vi "动力环境监测系统.vi"() -> ()   [LabVIEW 2016]
uses:
  DAM0404D/DAM0404D/DAM0404D.lvclass
  C:/Program Files (x86)/National Instruments/LabVIEW 2016/vi.lib/ActorFramework/Actor/Actor.lvclass
  DAM0404D/DAM0404D/DAM0404D.lvclass/DAM0404D.ctl
  <vilib>/ActorFramework/Message Enqueuer/Message Enqueuer.lvclass/Message Enqueuer.ctl
  DAM0404D/DAM0404D Messages/Write Coil Msg/Write Coil Msg.lvclass/Write Coil Msg.ctl
  <vilib>/ActorFramework/Message Enqueuer/Enqueue.vi
  <vilib>/ActorFramework/Stop Msg/Stop Msg.lvclass
  C:/Program Files (x86)/National Instruments/LabVIEW 2016/vi.lib/ActorFramework/Message/Message.lvclass
  DAM0404D/DAM0404D Messages/Close MB Msg/Close MB Msg.lvclass
  DAM0404D/DAM0404D Messages/Open MB Msg/Open MB Msg.lvclass
  DAM0404D/DAM0404D Messages/Write Coil Msg/Write Coil Msg.lvclass
  DAM0404D/DAM0404D Messages/Read sTA Msg/Read sTA Msg.lvclass
  <vilib>/ActorFramework/Message Priority Queue/Priority Enqueue.vi
  <vilib>/ActorFramework/Actor/Actor.lvclass
  <vilib>/Utility/config.llb/NI_LVConfig.lvlib
panel:
  in  "Log":string
  out "Busy":bool
  in  "Boolean":bool
  in  "断电":bool
  in  "通电":bool
  out "Array":bool[](array[boolean])
  in  "串口打开":bool
  in  "VISA resource name":refnum<visa-resource-name>
  # "254：9600"
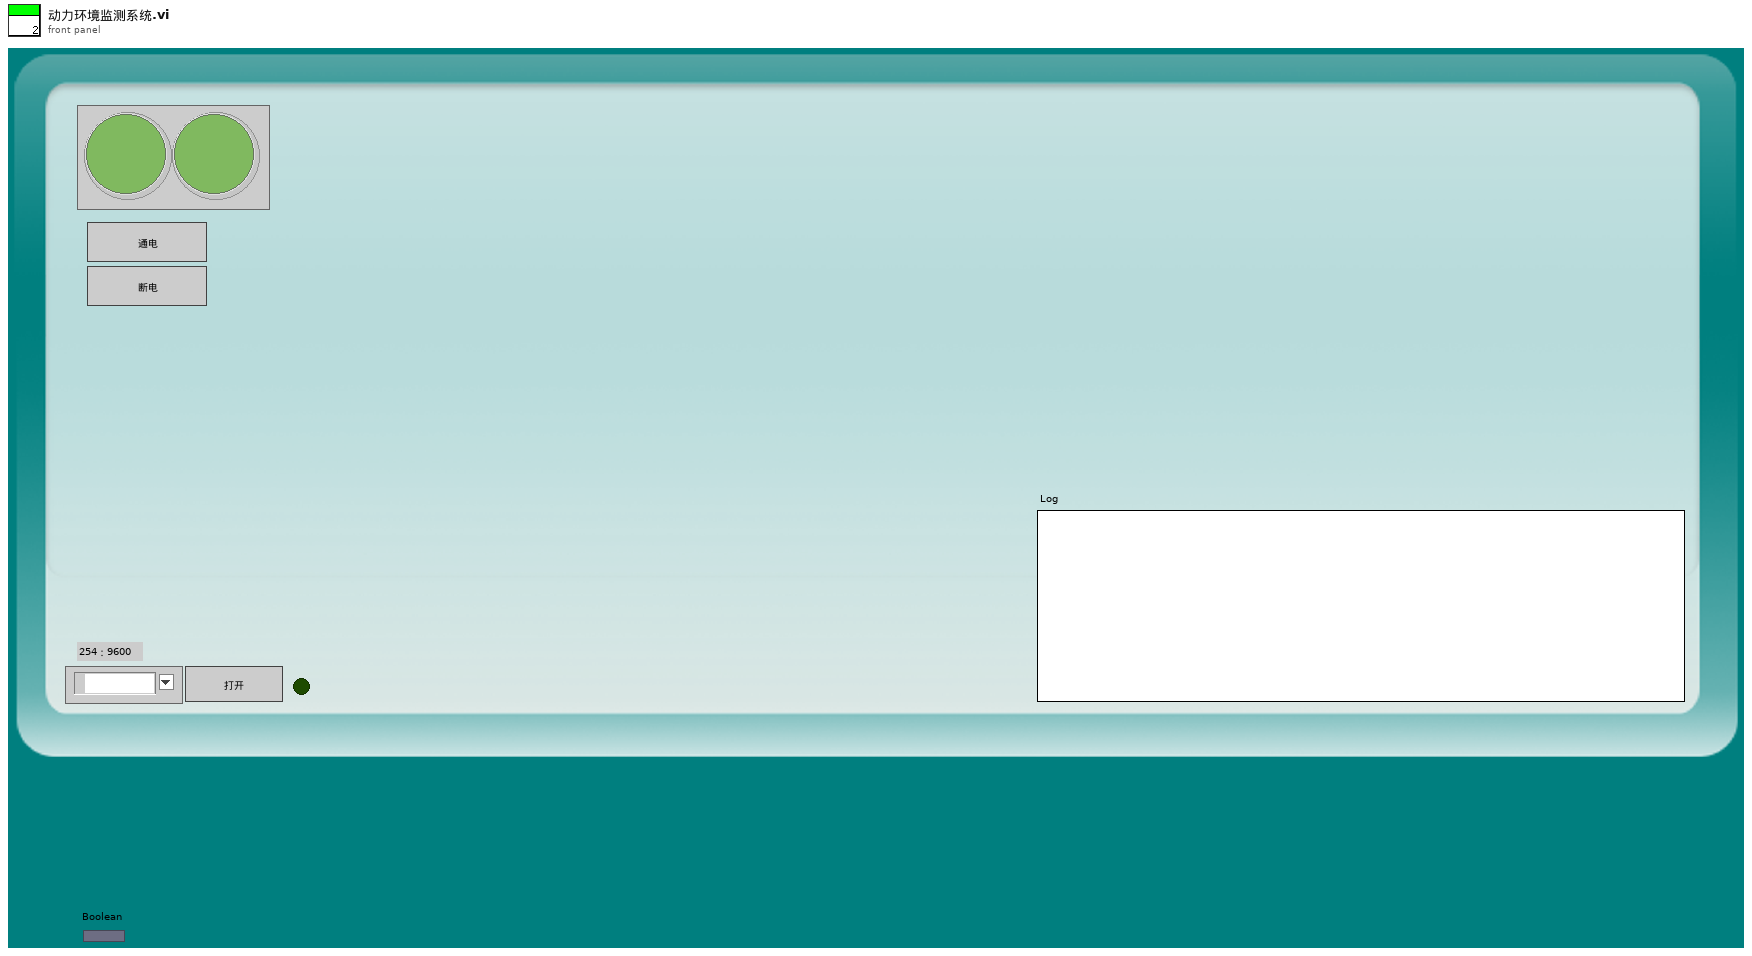
[diagram p1: front panel]
types:
  T1 = enum8{"Enabled", "Disabled", "Disabled and Grayed Out"}
  T2 = typedef "NI_LVConfig.lvlib/Config Data RefNum.ctl" = refnum<k1>
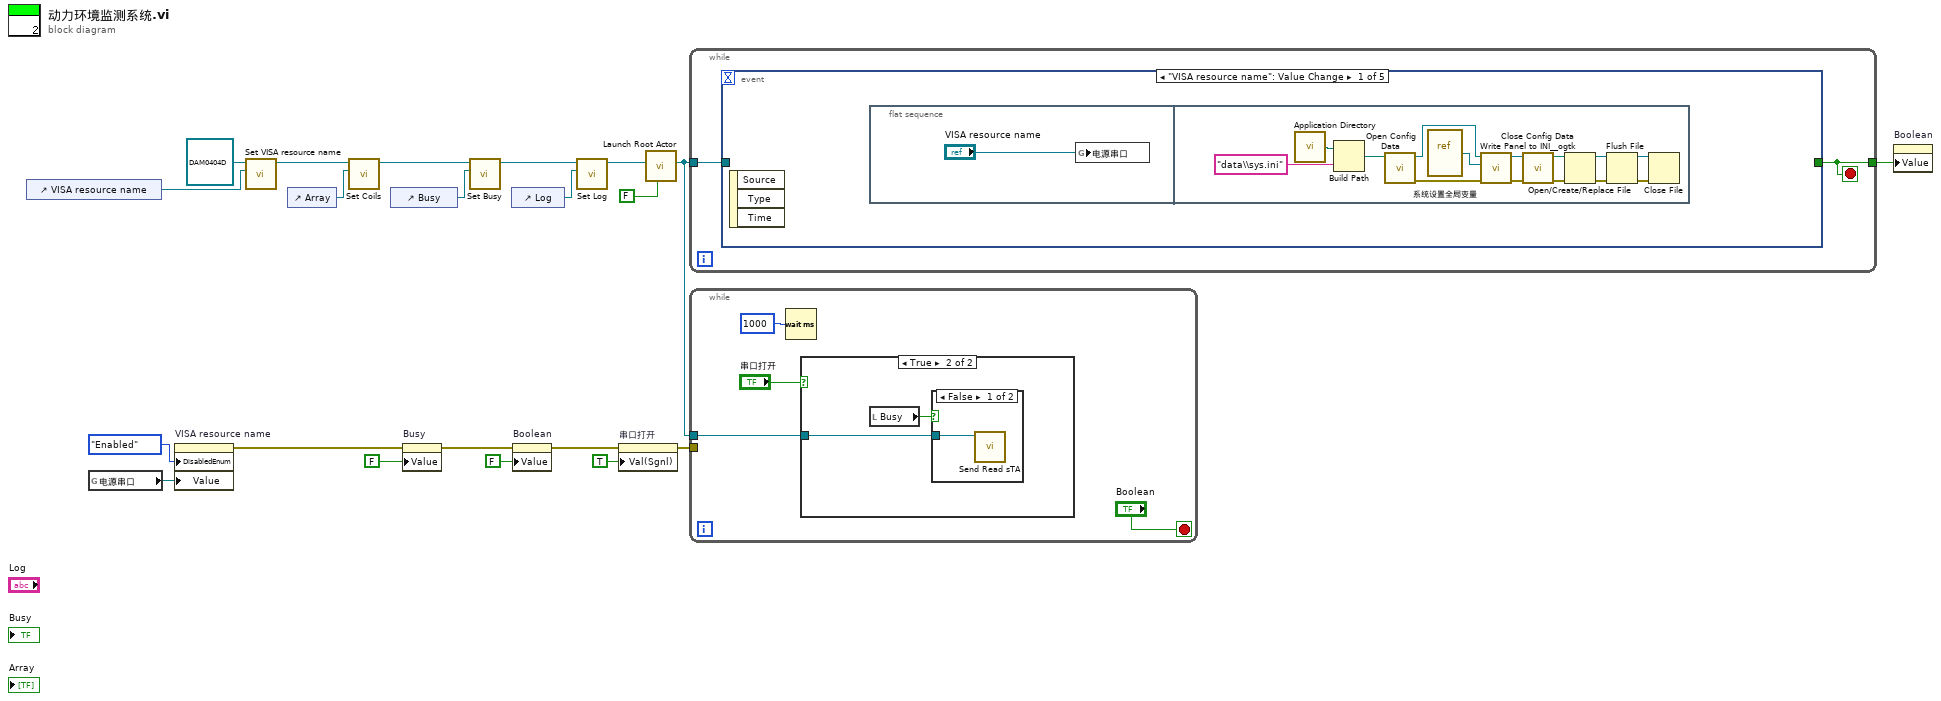
[diagram p0: block diagram]
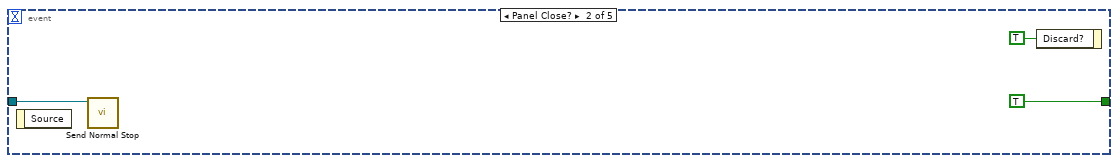
[diagram p4: hidden frame]
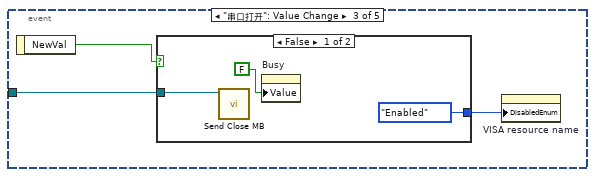
[diagram p5: hidden frame]
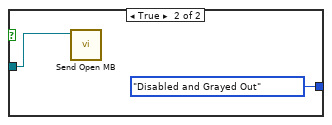
[diagram p6: hidden frame]
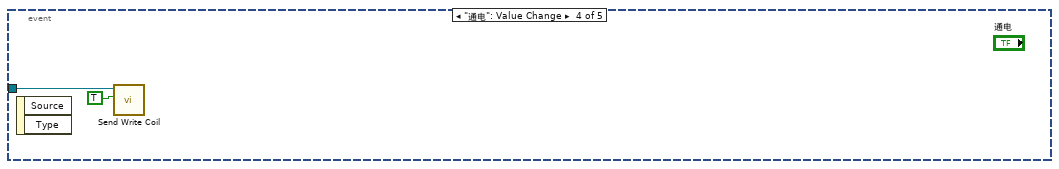
[diagram p7: hidden frame]
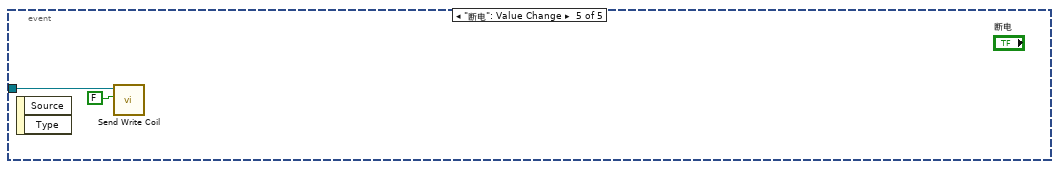
[diagram p8: hidden frame]
diagram:
  n1 = control-ref of="VISA resource name"() -> (w5:refnum<vi>)
  n2 = global read "系统设置全局变量.vi" "电源串口"() -> (w4:refnum<visa-resource-name>)
  n3 = property on="VISA resource name" class="VISAName"("DisabledEnum"=T1."Enabled" ("Disabled"), "Value"=w4) -> (error out=w10:errorcluster)  [unwired: 2 in, 1 out]
  n4 = call "Set VISA resource name.vi"("VISA resource name"=w5, "DAM0404D in"=refnum<class "DAM0404D.lvclass"> refnum ("DAM0404D.lvlib:DAM0404D.lvclass")) -> ("DAM0404D out"=w20:refnum<class "DAM0404D.lvclass">)  [unwired: 9 in]
  n5 = control-ref of="Array"() -> (w19:refnum<vi>)
  n6 = call "Set Coils.vi"("Coils"=w19, "DAM0404D in"=w20) -> ("DAM0404D out"=w14:refnum<class "DAM0404D.lvclass">)  [unwired: 9 in]
  n7 = control-ref of="Busy"() -> (w13:refnum<vi>)
  n8 = property on="Busy" class="Bool (strict)"(error in=w10, "Value"=FALSE ("Busy")) -> (error out=w12:errorcluster)  [unwired: 1 in, 1 out]
  n9 = call "Set Busy.vi"("Busy"=w13, "DAM0404D in"=w14) -> ("DAM0404D out"=w8:refnum<class "DAM0404D.lvclass">)  [unwired: 9 in]
  n10 = control-ref of="Log"() -> (w6:refnum<vi>)
  n11 = property on="Boolean" class="Bool (strict)"(error in=w12, "Value"=FALSE ("Boolean")) -> (error out=w3:errorcluster)  [unwired: 1 in, 1 out]
  n12 = call "Set Log.vi"("Log"=w6, "DAM0404D in"=w8) -> ("DAM0404D out"=w7:refnum<class "DAM0404D.lvclass">)  [unwired: 9 in]
  n13 = property on="串口打开" class="Bool (strict)"(error in=w3, "Val(Sgnl)"=TRUE ("Value (Signaling)")) -> (error out=w2:errorcluster)  [unwired: 1 in, 1 out]
  n14 = call <vilib>:"Launch Root Actor.vi"("Open Actor Core front panel? (F)"=FALSE, "Actor"=w7) -> ("Actor's Enqueuer"=w17:refnum<class "Message Enqueuer.lvclass">)  [unwired: 8 in, 1 out]
  n15 = while {
    tunnel: w17 -> [w23]
    tunnel: [w22] -> w18
    stop <- w22 stop-if-true
    n16 = event shown="[0] \"VISA resource name\": Value Change" {
      selector: _ -> [_ _ _ _ _]
      dyn-events: _ -> [_ _ _ _ _]
      timeout: _ -> [_ _ _ _ _]
      tunnel: [_ TRUE _ _ _] -> w22
      tunnel: w23 -> [_ w39 w44 w51 w53]
      event "VISA resource name": Value Change {
        n17 = event-data() -> ()  [unwired: 1 in, 3 out]
        n18 = flat-sequence {
          frame #0 {
            n19 = global write "系统设置全局变量.vi" "电源串口"("VISA resource name") -> ()
          }
          frame #1 {
            n20 = call <vilib>:"Application Directory.vi"() -> ("Application Directory"=w38:path)
            n21 = Build Path(base path=w38, name or relative path="data\\sys.ini" ("名称或相对路径")) -> (appended path=w36:path)
            n22 = call <vilib>:"Open Config Data.vi"("configuration file path"=w36) -> ("error out"=w32:errorcluster, "refnum"=w35:T2)  [unwired: 8 in, 1 out]
            n23 = vi-ref "系统设置全局变量.vi"() -> (w34:refnum<vi>)
            n24 = call <userlib>:"Write Panel to INI__ogtk.vi"("error in (no error)"=w32, "VI ref"=w34, "refnum"=w35) -> ("error out"=w31:errorcluster, "refnum out"=w33:T2)  [unwired: 7 in]
            n25 = call <vilib>:"Close Config Data.vi"("error in (no error)"=w31, "refnum"=w33) -> ("error out"=w26:errorcluster, "file path"=w25:path)  [unwired: 8 in]
            n26 = Open/Create/Replace File(file path (use dialog)=w25, error in=w26) -> (refnum out=w29:refnum<file>, error out=w30:errorcluster)  [unwired: 4 in, 1 out]
            n27 = Flush File(refnum=w29, error in=w30) -> (refnum out=w28:refnum<file>, error out=w27:errorcluster)
            n28 = Close File(refnum=w28, error in=w27) -> ()  [unwired: 2 out]
          }
        }
      }
      event Panel Close? {
        n29 = event-data() -> ()  [unwired: 1 in, 1 out]
        n30 = call <vilib>:"Send Normal Stop.vi"("Message Enqueuer"=w39) -> ()  [unwired: 10 in, 1 out]
        n31 = event-data("Discard?"=TRUE) -> ()  [unwired: 1 in, 1 out]
      }
      event "串口打开": Value Change {
        n32 = event-data() -> ("NewVal"=w43:bool)  [unwired: 1 in]
        n33 = case shown="False" w43 {
          tunnel: w44 -> [w46 w49]
          tunnel: [T1."Enabled" ("Disabled") T1."Disabled and Grayed Out" ("Disabled")] -> w42
          frame False {
            n34 = call "Send Close MB.vi"("Message Enqueuer"=w46) -> ()  [unwired: 9 in, 2 out]
            n35 = property on="Busy" class="Bool (strict)"("Value"=FALSE ("Busy")) -> ()  [unwired: 2 in, 2 out]
          }
          frame True {
            n36 = call "Send Open MB.vi"("Message Enqueuer"=w49) -> ()  [unwired: 9 in, 2 out]
          }
        }
        n37 = property on="VISA resource name" class="VISAName"("DisabledEnum"=w42) -> ()  [unwired: 2 in, 2 out]
      }
      event "通电": Value Change {
        n38 = event-data() -> ()  [unwired: 1 in, 2 out]
        n39 = call "Send Write Coil.vi"("Boolean"=TRUE, "Message Enqueuer"=w51) -> ()  [unwired: 8 in, 2 out]
      }
      event "断电": Value Change {
        n40 = event-data() -> ()  [unwired: 1 in, 2 out]
        n41 = call "Send Write Coil.vi"("Boolean"=FALSE, "Message Enqueuer"=w53) -> ()  [unwired: 8 in, 2 out]
      }
    }
  }
  n42 = while {
    tunnel: w17 -> [w55]
    tunnel: w2 -> [_]
    stop <- "Boolean" stop-if-true
    n43 = Wait (ms)(milliseconds to wait=u32 1000) -> ()  [unwired: 1 out]
    n44 = case shown="True" "串口打开" {
      tunnel: w55 -> [_ w59]
      frame False {
      }
      frame True {
        n45 = local read "Busy"() -> (w58:bool)
        n46 = case shown="False" w58 {
          tunnel: w59 -> [w60 _]
          frame False {
            n47 = call "Send Read sTA.vi"("Message Enqueuer"=w60) -> ()  [unwired: 9 in, 2 out]
          }
          frame True {
          }
        }
      }
    }
  }
  n48 = property on="Boolean" class="Bool (strict)"("Value"=w18) -> ()  [unwired: 2 in, 2 out]
